vi "Test Navigation API.vi"() -> ()   [LabVIEW 2020]
doc: "Navigation API Tester.\n\n<b>Note:</b> This VI was modified by the <b>Validate DQMH Module</b> tool to add the 'Show Main VI Diagram on Init' functionality included in DQMH 6.1.\n\n<b>Note:</b> This VI was modified by the <b>Validate DQMH Module</b> tool to upgrade its Error Reported event frame to use an improved mechanism for displaying error information.\n\n____\nHAMPEL SOFTWARE ENGINEERING v2.6.0 (2023-12-19 10:54)"
uses:
  Sub-VIs/Visibility options--enum.ctl
  <vilib>/Utility/error.llb/DialogType.ctl
  <vilib>/Hampel Software Engineering/HSE Logger/LogRecord/LogRecord.lvclass/LogRecord.ctl
  Navigation.lvlib
  Libraries/hse-libraries/Source/hse-dqmh/hse-dqmh.lvlib
  <vilib>/Hampel Software Engineering/HSE Logger/LogRecord/LogRecord.lvclass
  <vilib>/Hampel Software Engineering/HSE Logger/hse-logger.lvlib
panel:
  in  "Show Main VI Diagram on Init (F)":bool
  in  "Prepare":bool
  in  "Configure":bool
  in  "Control State":T1(ring)
  in  "DIS Control Name":string caption="Control Name"
  in  "Set Disabled State":bool
  in  "VIS Control Name":string caption="Control Name"
  in  "Visibility":T2
  in  "Set Visibility":bool
  in  "Select Listbox Element":bool
  in  "Select Row":i32
  out "Sub-Ctl OldVal":i32
  out "Sub-Ctl NewVal":i32
  out "Sub-Ctl Name":string
  out "Button Action":string
  out "Button Name":string
  in  "ListBox Name":string
  in  "Show Block Diagram":bool
  in  "Stop Module":bool
  in  "Start Module":bool
  in  "Hide Module Panel":bool
  in  "Show Module Panel":bool
  out "Status":string
  out "Module Running?":bool
  # "Button Pressed Events"
  # "Sub-Control Pressed Events"
  # "Set Visibility"
  # "Set Disabled State"
  # "Manipulate Sub-Controls (ListBoxes)"
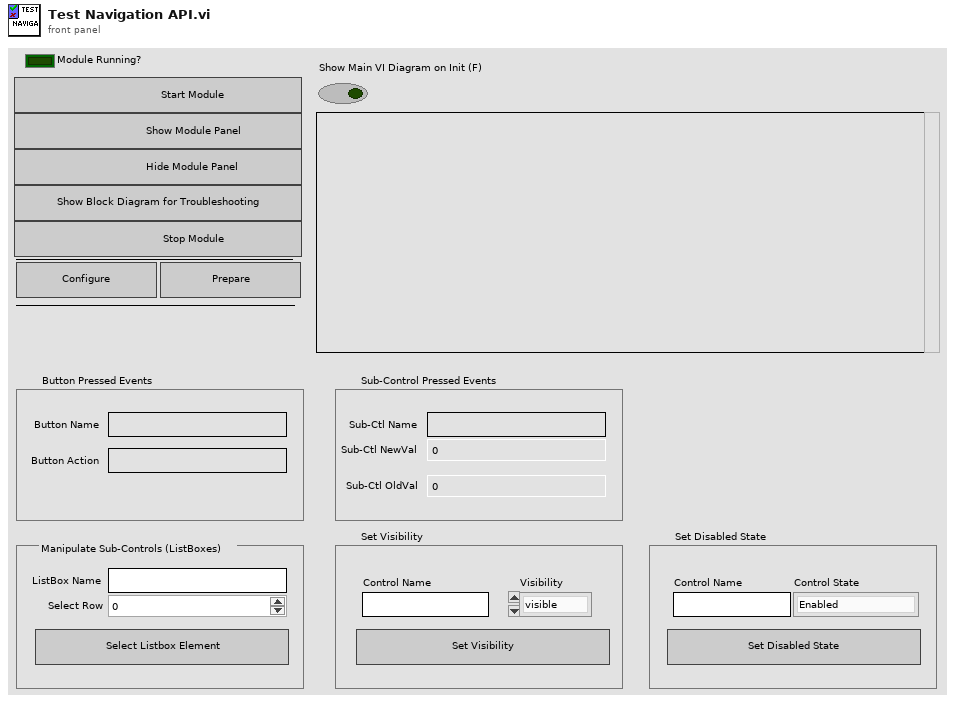
[diagram p1: front panel]
types:
  T1 = enum8{"Enabled", "Disabled", "Disabled and Grayed Out"}
  T2 = typedef "Navigation.lvlib/Visibility options--enum.ctl" = enum16{"visible", "hidden"}
  T3 = typedef "Navigation.lvlib/Broadcast Events--cluster.ctl" = cluster{"Module Did Init":refnum<user-event>, "Status Updated":refnum<user-event>, "Error Reported":refnum<user-event>, "Module Did Stop":refnum<user-event>, "Update Module Execution Status":refnum<user-event>, "Button Pressed":refnum<user-event>, "Sub-Control Pressed":refnum<user-event>, "System Message":refnum<user-event>}
  T4 = typedef "DialogType.ctl" = u16
  T5 = typedef "hse-dqmh.lvlib/System Message Source.ctl" = enum16{"module", "application", "network"}
  T6 = typedef "hse-logger.lvlib/LogLevel.ctl" = enum16{"DEBUG", "INFO", "WARNING", "ERROR", "CRITICAL"}
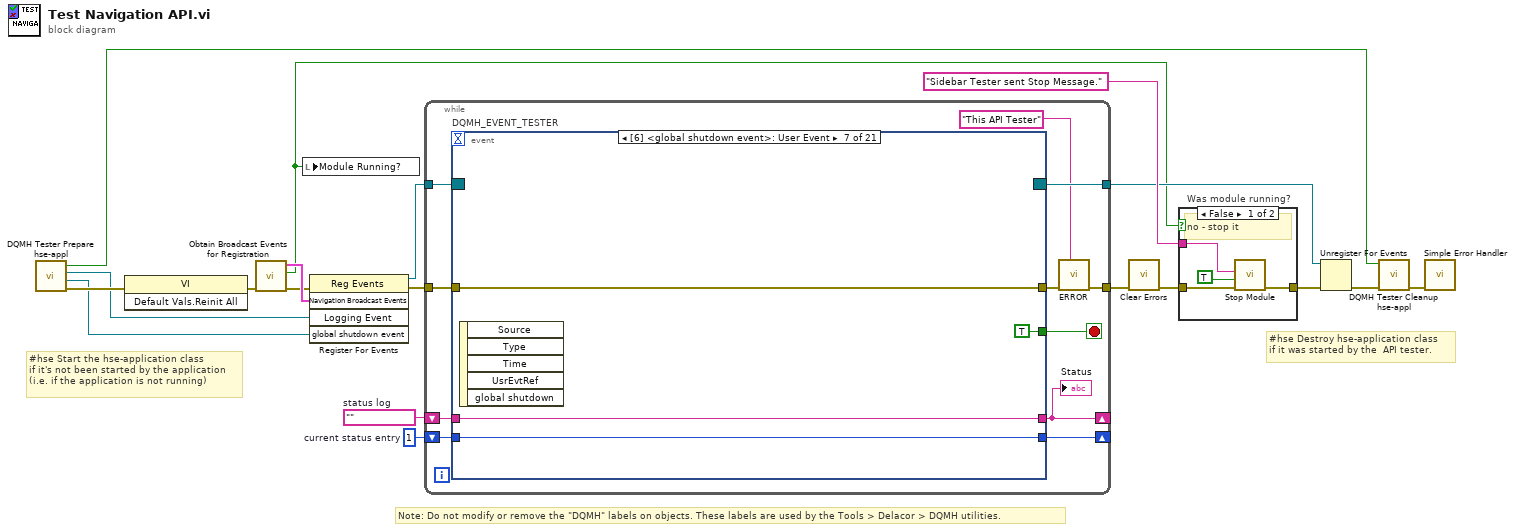
[diagram p0: block diagram]
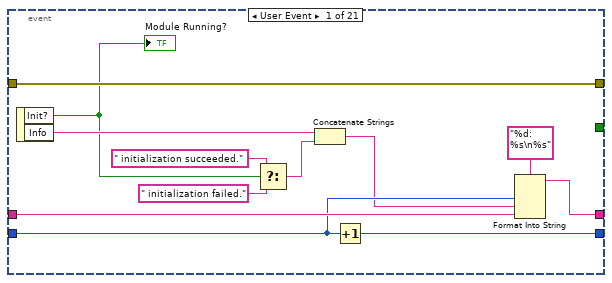
[diagram p3: hidden frame]
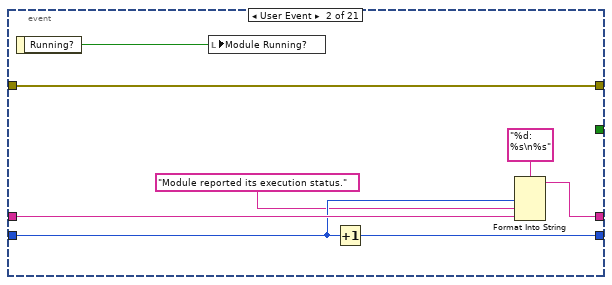
[diagram p4: hidden frame]
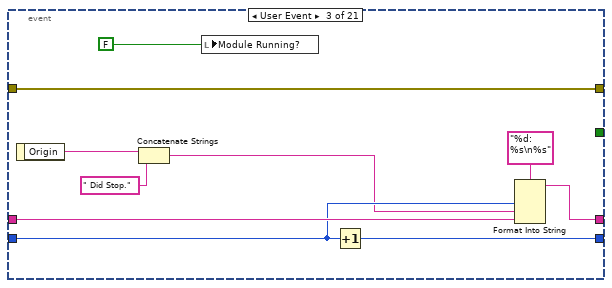
[diagram p5: hidden frame]
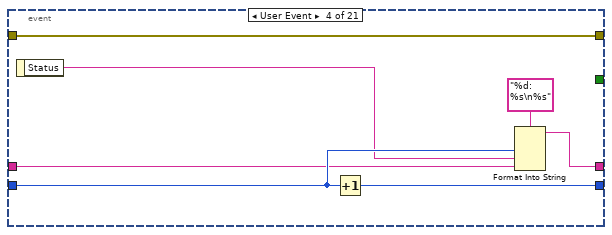
[diagram p6: hidden frame]
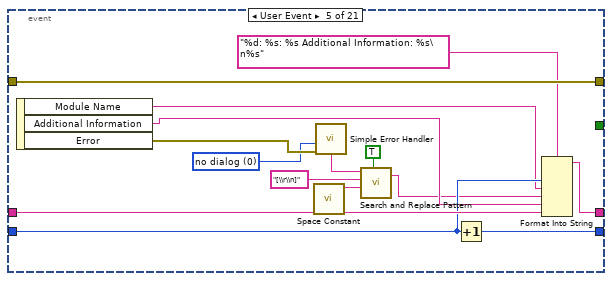
[diagram p7: hidden frame]
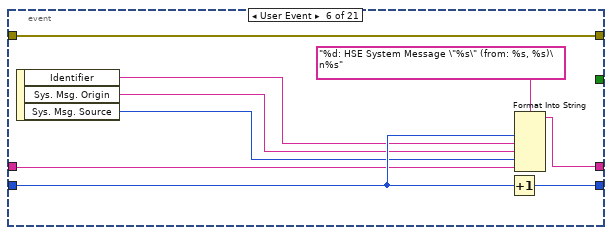
[diagram p8: hidden frame]
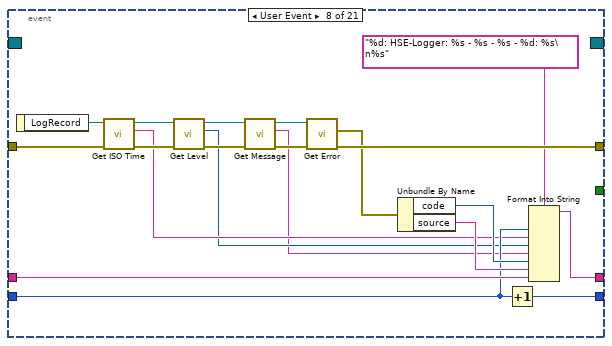
[diagram p9: hidden frame]
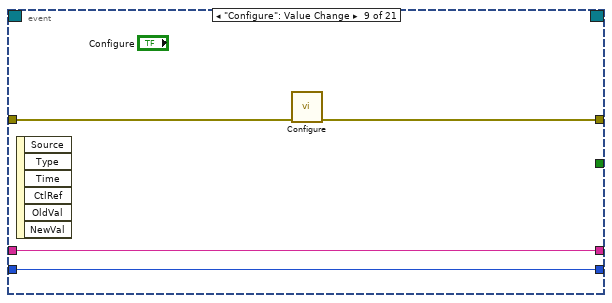
[diagram p10: hidden frame]
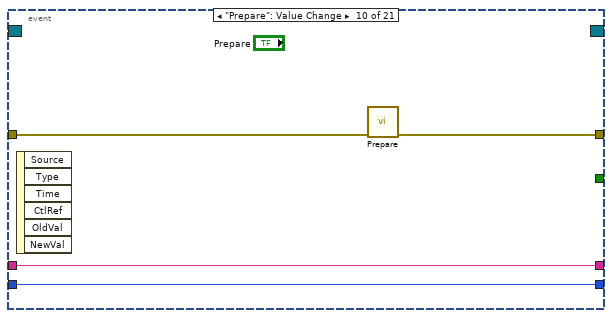
[diagram p11: hidden frame]
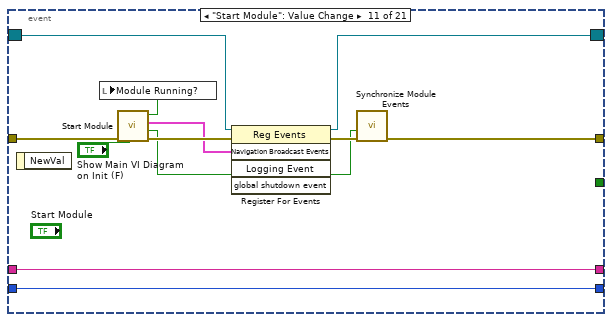
[diagram p12: hidden frame]
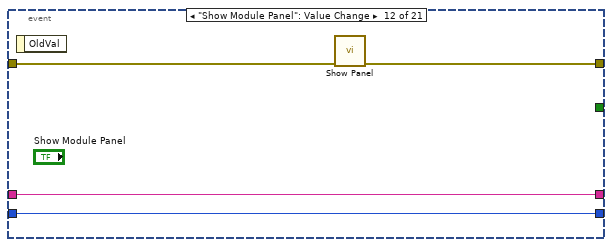
[diagram p13: hidden frame]
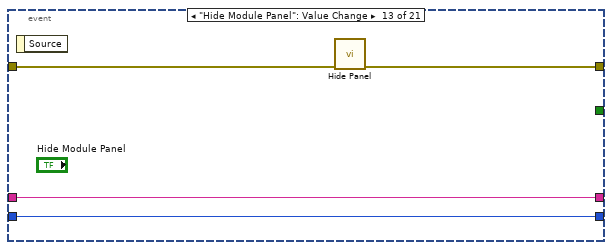
[diagram p14: hidden frame]
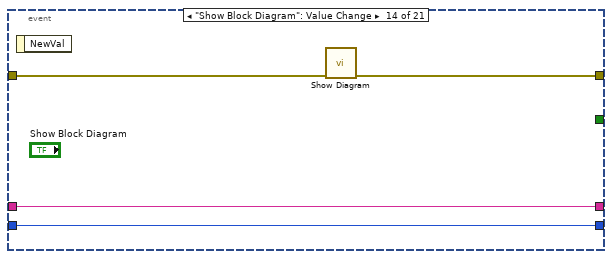
[diagram p15: hidden frame]
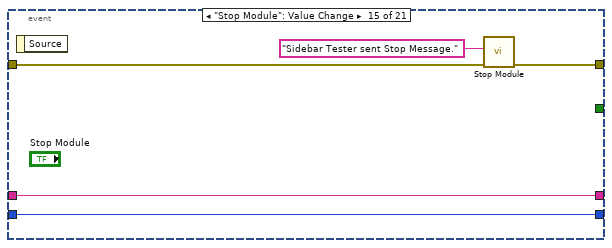
[diagram p16: hidden frame]
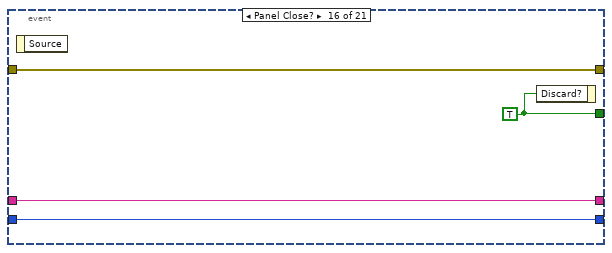
[diagram p17: hidden frame]
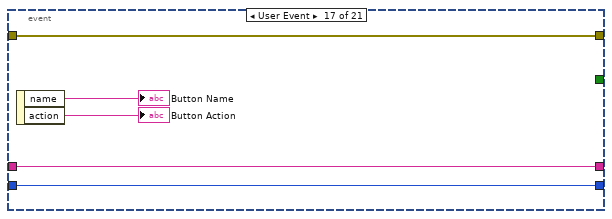
[diagram p18: hidden frame]
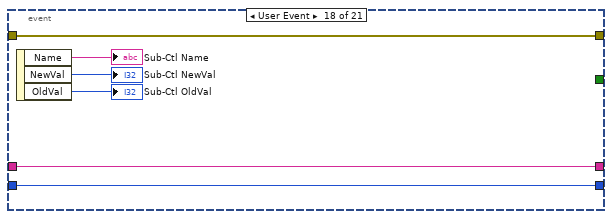
[diagram p19: hidden frame]
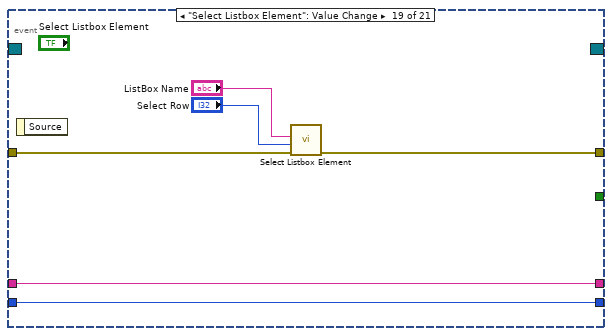
[diagram p20: hidden frame]
diagram:
  w16 = 1  # current status entry
  w17 = ""  # status log
  # "#hse Destroy hse-application class \nif it was started by the  API tester."
  # "#hse Start the hse-application class \nif it's not been started by the application\n(i.e. if the application is not running)"
  # "Note: Do not modify or remove the \"DQMH\" labels on objects. These labels are used by the Tools > Delacor > DQMH utilities."
  n1 = call "DQMH Tester Prepare hse-appl.vi"() -> ("error out"=w7:errorcluster, "global shutdown event"=w1:refnum<user-event>, "Logging Event"=w6:refnum<user-event>, "Started?"=w4:bool)  [unwired: 8 in]
  n2 = invoke class="VI" method="Default Vals.Reinit All"(error in=w7) -> (error out=w9:errorcluster)  [unwired: 2 in, 2 out]
  n3 = call "Obtain Broadcast Events for Registration.vi"("error in (no error)"=w9) -> ("error out"=w8:errorcluster, "Already running?"=w3:bool, "Navigation Broadcast Events"=w14:T3)  [unwired: 8 in]
  n4 = local write "Module Running?"(w3) -> ()
  n5 = register-events(error in=w8, w14, w6, w1) -> (reference out=w13:refnum<event-registration>, error out=w15:errorcluster)  [unwired: 1 in]
  n6 = while {
    tunnel: w13 -> [w30]
    tunnel: [w21] -> w10
    shift-right: [w26] -> _
    shift-left: w17 -> [w28]
    shift-right: [w27] -> _
    shift-left: w16 -> [w29]
    tunnel: w15 -> [w25]
    tunnel: [w24] -> w12
    stop <- w22 stop-if-true
    n7 = event "DQMH_EVENT_TESTER" shown="[6] <global shutdown event>: User Event" {
      selector: w30 -> [_ _ _ _ _ _ _ _ _ _ w129 _ _ _ _ _ _ _ _ _ _]
      dyn-events: [_ _ _ _ _ _ _ _ _ _ w128 _ _ _ _ _ _ _ _ _ _] -> w24
      timeout: _ -> [_ _ _ _ _ _ _ _ _ _ _ _ _ _ _ _ _ _ _ _ _]
      tunnel: [_ _ _ _ _ _ TRUE ("Discard?") _ _ _ _ _ _ _ _ w156 _ _ _ _ _] -> w22
      tunnel: [w42 w44 w51 w61 w82 w91 w95 w115 w116 w120 w125 w139 w143 w144 w150 w153 w161 w167 w170 w176 w182] -> w23
      tunnel: w29 -> [w39 w48 w58 w64 w79 w89 w93 w101 w118 w122 w132 w137 w141 w145 w151 w154 w159 w165 w171 w177 w183]
      tunnel: w28 -> [w40 w49 w59 w63 w81 w84 w94 w103 w119 w123 w133 w138 w142 w146 w152 w155 w160 w166 w172 w178 w184]
      tunnel: [w37 w46 w56 w65 w80 w83 w94 w102 w119 w123 w133 w138 w142 w146 w152 w155 w160 w166 w172 w178 w184] -> w26
      tunnel: [w38 w47 w57 w67 w78 w88 w93 w100 w118 w122 w132 w137 w141 w145 w151 w154 w159 w165 w171 w177 w183] -> w27
      tunnel: w25 -> [w42 w44 w51 w61 w82 w91 w95 w108 w117 w121 w127 w136 w140 w147 w148 w153 w161 w167 w173 w179 w185]
      event User Event {
        n8 = event-data() -> ("Init?"=w34:bool, "Info"=w36:string)  [unwired: 1 in]
        "Module Running?" <- w34
        n9 = Select(t=" initialization succeeded.", s=w34, f=" initialization failed.") -> (s? t:f=w31:string)
        n10 = Concatenate Strings(w36, w31) -> (w35:string)
        n11 = Increment(x=w39) -> (x+1=w38:i32)
        n12 = Format Into String(format string="%d: %s\n%s", w39, w35, w40) -> (resulting string=w37:string)  [unwired: 2 in, 1 out]
      }
      event User Event {
        n13 = event-data() -> ("Running?"=w43:bool)  [unwired: 1 in]
        n14 = local write "Module Running?"(w43) -> ()
        n15 = Increment(x=w48) -> (x+1=w47:i32)
        n16 = Format Into String(format string="%d: %s\n%s", w48, "Module reported its execution status.", w49) -> (resulting string=w46:string)  [unwired: 2 in, 1 out]
      }
      event User Event {
        n17 = event-data() -> ("Origin"=w55:string)  [unwired: 1 in]
        n18 = Concatenate Strings(w55, " Did Stop.") -> (w54:string)
        n19 = local write "Module Running?"(FALSE ("Module Did Init?")) -> ()
        n20 = Increment(x=w58) -> (x+1=w57:i32)
        n21 = Format Into String(format string="%d: %s\n%s", w58, w54, w59) -> (resulting string=w56:string)  [unwired: 2 in, 1 out]
      }
      event User Event {
        n22 = event-data() -> ("Status"=w62:string)  [unwired: 1 in]
        n23 = Increment(x=w64) -> (x+1=w67:i32)
        n24 = Format Into String(format string="%d: %s\n%s", w64, w62, w63) -> (resulting string=w65:string)  [unwired: 2 in, 1 out]
      }
      event User Event {
        w74 = T4 0 items=["no dialog", "OK message", "continue or stop message", "OK message + warnings", "continue/stop + warnings"] ("type of dialog (OK msg:1)")
        n25 = event-data() -> ("Module Name"=w75:string, "Additional Information"=w76:string, "Error"=w77:errorcluster)  [unwired: 1 in]
        n26 = call <vilib>:"Space Constant.vi"() -> ("String"=w70:string)
        n27 = call <vilib>:"Simple Error Handler.vi"("type of dialog (OK msg:1)"=w74, "error in (no error)"=w77) -> ("message"=w73:string)  [unwired: 3 in, 4 out]
        n28 = call <vilib>:"Search and Replace Pattern.vi"("string"=w73, "regular expression (\"\")"="[\\r\\n]" ("regular expression (\"\")"), "replace string (\"\")"=w70, "replace all? (F)"=TRUE ("replace all CR/LF with spaces")) -> ("result string"=w72:string)  [unwired: 1 in, 1 out]
        n29 = Increment(x=w79) -> (x+1=w78:i32)
        n30 = Format Into String(format string="%d: %s: %s Additional Information: %s\n%s", w79, w75, w72, w76, w81) -> (resulting string=w80:string)  [unwired: 2 in, 1 out]
      }
      event User Event {
        n31 = event-data() -> ("Identifier"=w87:string, "Sys. Msg. Origin"=w86:string, "Sys. Msg. Source"=w85:T5)  [unwired: 1 in]
        n32 = Increment(x=w89) -> (x+1=w88:i32)
        n33 = Format Into String(format string="%d: HSE System Message \"%s\" (from: %s, %s)\n%s", w89, w87, w86, w85, w84) -> (resulting string=w83:string)  [unwired: 2 in, 1 out]
      }
      event User Event {
        n34 = event-data() -> ()  [unwired: 1 in, 5 out]
      }
      event User Event {
        n35 = event-data() -> ("LogRecord"=w107:refnum<class "LogRecord.lvclass">)  [unwired: 1 in]
        n36 = call <vilib>:"Get ISO Time.vi"("error in"=w108, "LogRecord in"=w107) -> ("error out"=w114:errorcluster, "ISO Time"=w98:string, "LogRecord out"=w113:refnum<class "LogRecord.lvclass">)  [unwired: 7 in]
        n37 = call <vilib>:"Get Level.vi"("error in"=w114, "LogRecord in"=w113) -> ("error out"=w111:errorcluster, "Level"=w97:T6, "LogRecord out"=w112:refnum<class "LogRecord.lvclass">)  [unwired: 7 in]
        n38 = call <vilib>:"Get Message.vi"("error in"=w111, "LogRecord in"=w112) -> ("error out"=w109:errorcluster, "Message"=w96:string, "LogRecord out"=w110:refnum<class "LogRecord.lvclass">)  [unwired: 7 in]
        n39 = call <vilib>:"Get Error.vi"("error in"=w109, "LogRecord in"=w110) -> ("error out"=w115:errorcluster, "Error"=w99:errorcluster)  [unwired: 7 in, 1 out]
        n40 = Unbundle By Name(w99) -> ("code"=w105:i32, "source"=w104:string)
        n41 = Increment(x=w101) -> (x+1=w100:i32)
        n42 = Format Into String(format string="%d: HSE-Logger: %s - %s - %s - %d: %s\n%s", w101, w98, w97, w96, w105, w104, w103) -> (resulting string=w102:string)  [unwired: 2 in, 1 out]
      }
      event "Configure": Value Change {
        n43 = event-data() -> ()  [unwired: 1 in, 6 out]
        n44 = call "Configure.vi"("error in (no error)"=w117) -> ("error out"=w116:errorcluster)  [unwired: 10 in]
      }
      event "Prepare": Value Change {
        n45 = event-data() -> ()  [unwired: 1 in, 6 out]
        n46 = call "Prepare.vi"("error in (no error)"=w121) -> ("error out"=w120:errorcluster)  [unwired: 10 in]
      }
      event "Start Module": Value Change {
        n47 = event-data() -> ()  [unwired: 1 in, 1 out]
        n48 = call "Start Module.vi"("Show Main VI Diagram on Init (F)"="Show Main VI Diagram on Init (F)", "error in (no error)"=w127) -> ("error out"=w134:errorcluster, "Wait for Event Sync?"=w131:bool, "Navigation Broadcast Events"=w130:T3, "Module Was Already Running?"=w126:bool)  [unwired: 6 in]
        n49 = local write "Module Running?"(w126) -> ()
        n50 = register-events(reference=w129, error in=w134, w130) -> (reference out=w128:refnum<event-registration>, error out=w135:errorcluster)  [unwired: 2 in]
        n51 = call "Synchronize Module Events.vi"("error in (no error)"=w135, "Wait for Event Sync?"=w131) -> ("error out"=w125:errorcluster)  [unwired: 9 in]
      }
      event "Show Module Panel": Value Change {
        n52 = event-data() -> ()  [unwired: 1 in, 1 out]
        n53 = call "Show Panel.vi"("error in (no error)"=w136) -> ("error out"=w139:errorcluster)  [unwired: 10 in]
      }
      event "Hide Module Panel": Value Change {
        n54 = event-data() -> ()  [unwired: 1 in, 1 out]
        n55 = call "Hide Panel.vi"("error in (no error)"=w140) -> ("error out"=w143:errorcluster)  [unwired: 10 in]
      }
      event "Show Block Diagram": Value Change {
        n56 = event-data() -> ()  [unwired: 1 in, 1 out]
        n57 = call "Show Diagram.vi"("error in (no error)"=w147) -> ("error out"=w144:errorcluster)  [unwired: 10 in]
      }
      event "Stop Module": Value Change {
        n58 = event-data() -> ()  [unwired: 1 in, 1 out]
        n59 = call "Stop Module.vi"("error in (no error)"=w148, "Origin"="Sidebar Tester sent Stop Message.") -> ("error out"=w150:errorcluster)  [unwired: 9 in]
      }
      event Panel Close? {
        w156 = TRUE ("Discard?")
        n60 = event-data() -> ()  [unwired: 1 in, 1 out]
        n61 = event-data("Discard?"=w156) -> ()  [unwired: 1 in, 1 out]
      }
      event User Event {
        n62 = event-data() -> ("name"=→"Button Name":string, "action"=→"Button Action":string)  [unwired: 1 in]
      }
      event User Event {
        n63 = event-data() -> ("Name"=→"Sub-Ctl Name":string, "NewVal"=→"Sub-Ctl NewVal":i32, "OldVal"=→"Sub-Ctl OldVal":i32)  [unwired: 1 in]
      }
      event "Select Listbox Element": Value Change {
        n64 = event-data() -> ()  [unwired: 1 in, 1 out]
        n65 = call "Select Listbox Element.vi"("error in (no error)"=w173, "Index"="Select Row", "Name"="ListBox Name") -> ("error out"=w170:errorcluster)  [unwired: 8 in]
      }
      event "Set Visibility": Value Change {
        n66 = event-data() -> ()  [unwired: 1 in, 1 out]
        n67 = call "Set Visibility.vi"("error in (no error)"=w179, "Visibility"="Visibility", "Control Name"="VIS Control Name") -> ("error out"=w176:errorcluster)  [unwired: 8 in]
      }
      event "Set Disabled State": Value Change {
        n68 = event-data() -> ()  [unwired: 1 in, 1 out]
        n69 = call "Set Disabled State.vi"("error in (no error)"=w185, "Control State"="Control State", "Control Name"="DIS Control Name") -> ("error out"=w182:errorcluster)  [unwired: 8 in]
      }
    }
    "Status" <- w26
    n70 = call <vilib>:"ERROR.vi"("Message"="This API Tester" ("Origin"), "error in"=w23) -> ("error out"=w21:errorcluster)  [unwired: 9 in]
  }
  n71 = call <vilib>:"Clear Errors.vi"("error in (no error)"=w10) -> ("error out"=w11:errorcluster)  [unwired: 5 in, 1 out]
  n72 = case "Was module running?" shown="False" w3 {
    tunnel: [w189 w190] -> w19
    tunnel: "Sidebar Tester sent Stop Message." ("Origin") -> [w188 _]
    tunnel: w11 -> [w186 w190]
    frame False {
      # "no - stop it"
      n73 = call "Stop Module.vi"("error in (no error)"=w186, "Wait for Module to Stop? (F)"=TRUE ("Wait for Module to stop?"), "Origin"=w188) -> ("error out"=w189:errorcluster)  [unwired: 8 in]
    }
    frame True {
      # "Yes - do nothing"
    }
  }
  n74 = Unregister For Events(event registration refnum=w12, error in=w19) -> (error out=w5:errorcluster)
  n75 = call "DQMH Tester Cleanup hse-appl.vi"("error in"=w5, "Stop?"=w4) -> ("error out"=w2:errorcluster)  [unwired: 9 in]
  n76 = call <vilib>:"Simple Error Handler.vi"("error in (no error)"=w2) -> ()  [unwired: 4 in, 5 out]
